vi "Main.vi"(7 "Event Sources":T1, 8 "error in":errorcluster, 9 "Folder names":string[](array[string])=["StaARx#[PLC]StaATesterRxSignals", "StaATx#[PLC]StaATesterTxSignals"], 10 "Sequence Context In":refnum<k7>, 11 "PostUUT In":refnum<class "PostUUT.lvclass">) -> (0 "error out":errorcluster, 3 "OPC UA Out":refnum<class "PostUUT.lvclass">, 5 "Station":string)   [LabVIEW 2021, in "PostUUT.lvclass"]
uses:
  PostUUT.lvclass
  Controls/Rx PostUUT.ctl
  Controls/Tx PostUUT.ctl
  PostUUT.lvclass/PostUUT.ctl
  <vilib>/addons/TestStand/_TSUtility.llb/TestStand - Get Property Value (Number {Signed 32-bit Integer}).vi
  OPC UA/OPC UA.lvclass
panel:
  out "Connect?":bool
  in  "Tx PostUUT":T2={"ResultsReady"=TRUE, "Results"=0, "ElapsedTime"=0, "TimeCompleted"=[], "Fault"=FALSE, "Timeout"=FALSE}
  out "Rx PostUUT":T3
  out "State":string="OPC UA.lvclass"
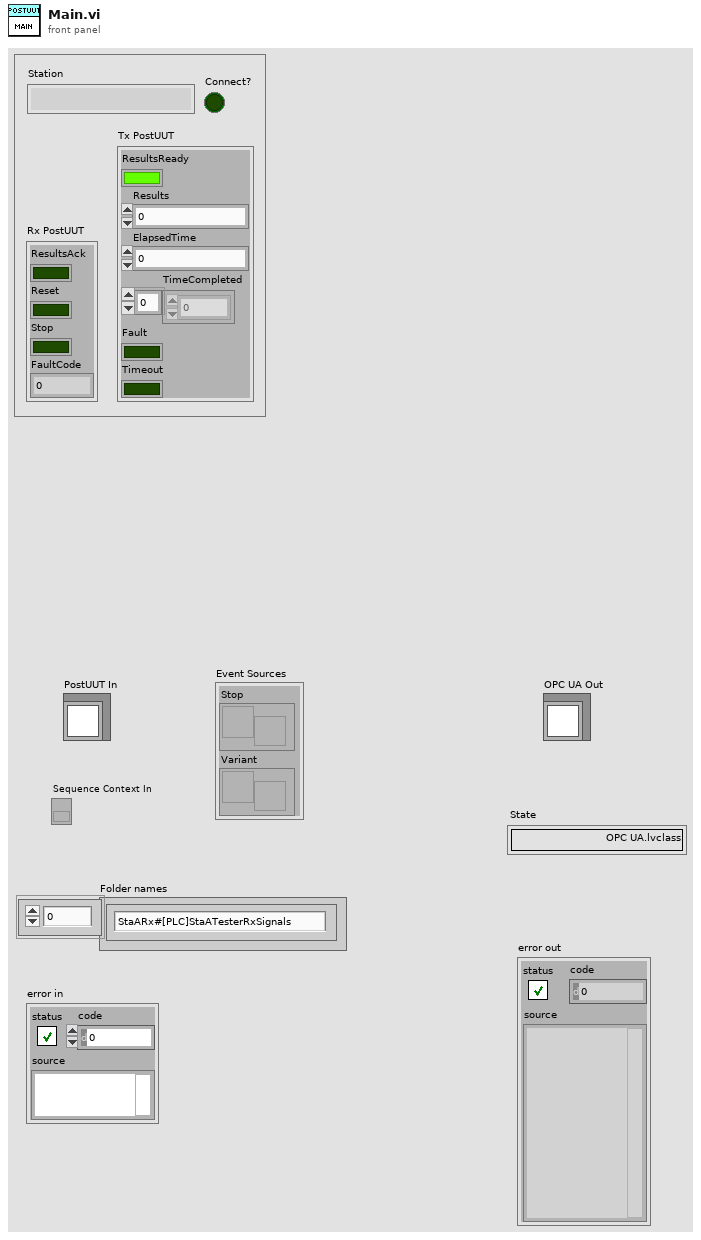
[diagram p1: front panel]
types:
  T1 = cluster{"Stop":refnum<user-event>, "Variant":refnum<user-event>}
  T2 = typedef "PostUUT.lvclass/Tx PostUUT.ctl" = cluster{"ResultsReady":bool, "Results":i32, "ElapsedTime":i32, "TimeCompleted":i32[], "Fault":bool, "Timeout":bool}
  T3 = typedef "PostUUT.lvclass/Rx PostUUT.ctl" = cluster{"ResultsAck":bool, "Reset":bool, "Stop":bool, "FaultCode":u32}
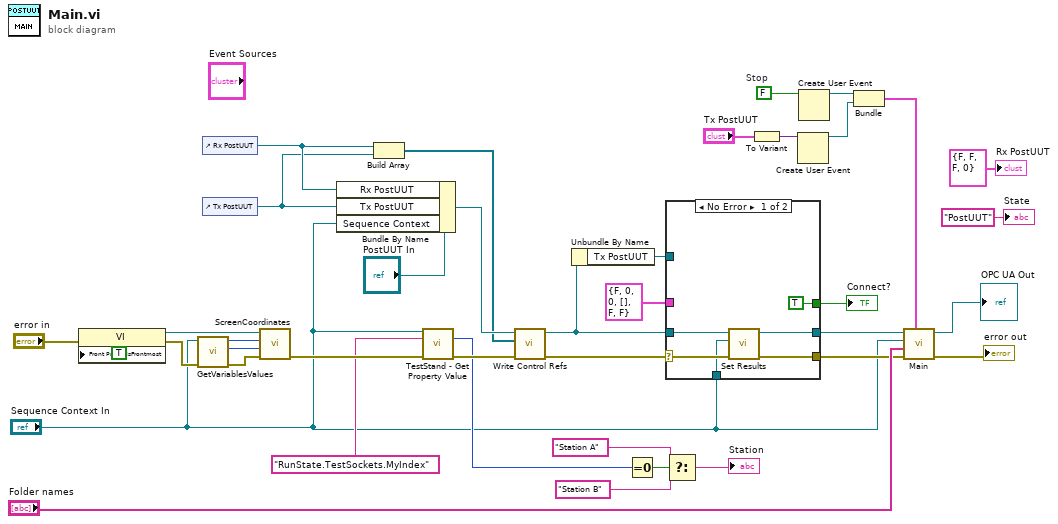
[diagram p0: block diagram]
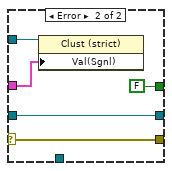
[diagram p2: hidden frame]
diagram:
  w21 = FALSE  # Stop
  n1 = property class="VI"(error in="error in", "Front Panel.IsFrontmost"=TRUE ("Front Panel Window:Is Frontmost")) -> (reference out=w13:refnum<vi>, error out=w11:errorcluster)  [unwired: 1 in]
  n2 = call "GetVariablesValues.vi"("error in (no error)"=w11, "Sequence Context In"="Sequence Context In") -> ("error out (no error)"=w12:errorcluster, "LeftCoordinates"=w15:i16, "TopCoordinates"=w14:i16)  [unwired: 6 in, 1 out]
  n3 = control-ref of="Rx PostUUT"() -> (w30:refnum<vi>)
  n4 = control-ref of="Tx PostUUT"() -> (w29:refnum<vi>)
  n5 = call "ScreenCoordinates.vi"("error in (no error)"=w12, "Left Coordinate"=w15, "Top Coordinate"=w14, "ThisVI"=w13) -> ("error out"=w16:errorcluster)  [unwired: 6 in, 1 out]
  n6 = Bundle By Name(cluster="PostUUT In", "Rx PostUUT"=w30, "Tx PostUUT"=w29, "Sequence Context"="Sequence Context In") -> (w28:refnum<class "PostUUT.lvclass">)
  n7 = Build Array(w30, w29) -> (w27:refnum<vi>[])
  n8 = call-poly <vilib>:"TestStand - Get Property Value.vi"("Sequence Context In"="Sequence Context In", "Lookup String"="RunState.TestSockets.MyIndex", "error in (no error)"=w16) -> ("Value"=w3:i32, "error out"=w8:errorcluster)  [unwired: 10 in, 1 out]
  n9 = call-dynamic "Write Control Refs.vi"("error in (no error)"=w8, "Ctl Refs"=w27, "OPC UA in"=w28) -> ("error out"=w26:errorcluster, "OPC UA out"=w23:refnum<class "PostUUT.lvclass">)  [unwired: 7 in]
  n10 = Unbundle By Name(w23) -> ("Tx PostUUT"=w35:refnum<vi>)
  n11 = Equal To 0?(x=w3) -> (x = 0?=w4:bool)
  n12 = case shown="No Error" w26 {
    selector: w26 -> [w42 w46]
    tunnel: w23 -> [w45 w50]
    tunnel: [w44 w50] -> w18
    tunnel: w35 -> [_ w49]
    tunnel: T2 {"ResultsReady"=FALSE, "Results"=0, "ElapsedTime"=0, "TimeCompleted"=[], "Fault"=FALSE, "Timeout"=FALSE} ("Value (Signaling)") -> [_ w48]
    tunnel: [TRUE ("Connect?") FALSE ("Connect?")] -> w31
    tunnel: [w41 w46] -> w17
    tunnel: "Sequence Context In" -> [w40 _]
    frame No Error {
      n13 = call "Set Results.vi"("error in (no error)"=w42, "Sequence Context"=w40, "PostUUT in"=w45) -> ("error out"=w41:errorcluster, "PostUUT out"=w44:refnum<class "PostUUT.lvclass">)  [unwired: 7 in]
    }
    frame Error {
      n14 = property class="Clust (strict)"(reference=w49, "Val(Sgnl)"=w48) -> ()  [unwired: 1 in, 2 out]
    }
  }
  "Connect?" <- w31
  n15 = Select(t="Station A" ("initial string"), s=w4, f="Station B" ("initial string")) -> (s? t:f=→"Station":string)
  n16 = To Variant(anything="Tx PostUUT") -> (Variant=w38:variant)
  n17 = Create User Event(user event datatype=w38) -> (user event=w20:refnum<user-event>)  [unwired: 1 in, 1 out]
  n18 = Create User Event(user event datatype=w21) -> (user event=w22:refnum<user-event>)  [unwired: 1 in, 1 out]
  n19 = Bundle("Stop"=w22, "Variant"=w20) -> (w19:T1)  [unwired: 1 in]
  n20 = call-parent "Main.vi"("Event Sources"=w19, "error in"=w17, "Folder names"="Folder names", "Sequence Context In"="Sequence Context In", "OPC UA In"=w18) -> ("error out"=→"error out":errorcluster, "OPC UA Out"=→"OPC UA Out":refnum<class "PostUUT.lvclass">)  [unwired: 4 in, 1 out]
  "State" <- "PostUUT" ("State")
  "Rx PostUUT" <- T3 {"ResultsAck"=FALSE, "Reset"=FALSE, "Stop"=FALSE, "FaultCode"=0} ("Rx PostUUT")
